vi "McP789A-Move-Server v0.80.vi"(5 "Initializing MCP":bool, 6 "Change Counter Position Manually":bool, 7 "error in":errorcluster, 8 "Unit":u8(ring)=1 items=["Point #", "nm", "eV", "meV", "cm-1"], 9 "New Position":dbl=600.0 min=0.0 max=100000.0 format="%.3f", 10 "Grating Density":enum16{"150", "300", "600", "1200", "1800"}(ring)=enum."1800") -> (0 "error out":errorcluster={"status"=TRUE, "code"=65, "source"="McP Timeout"}, 1 "Final Stepper Position":i32=-1000000, 2 "Final Wavelenth (nm)":dbl=222.0 format="%.2f", 3 "Final CounterReading":dbl=10000.0 min=0.0 max=26000.0 format="%.2f", 4 "Final Position":dbl=222.0 format="%.2f")   [LabVIEW 2020]
doc: "McPherson 789A-3 controller Vi to control McPherson 2075 spectrometer through serial port. If running directly, you need to initialize the serial port and the spectrometer. During this process, if the scan velocity returns to be 0, the program is suspended. You need to change the velocity manually to unblock."
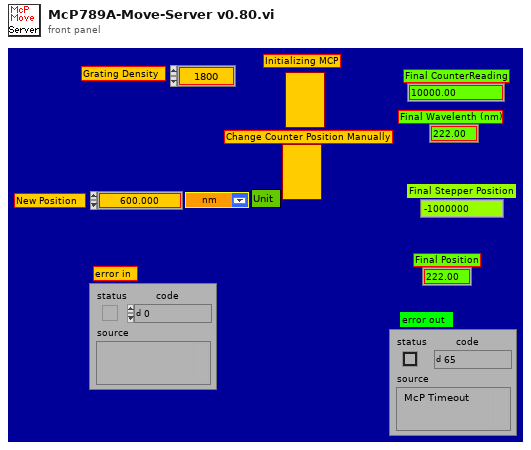
[diagram p1: front panel]
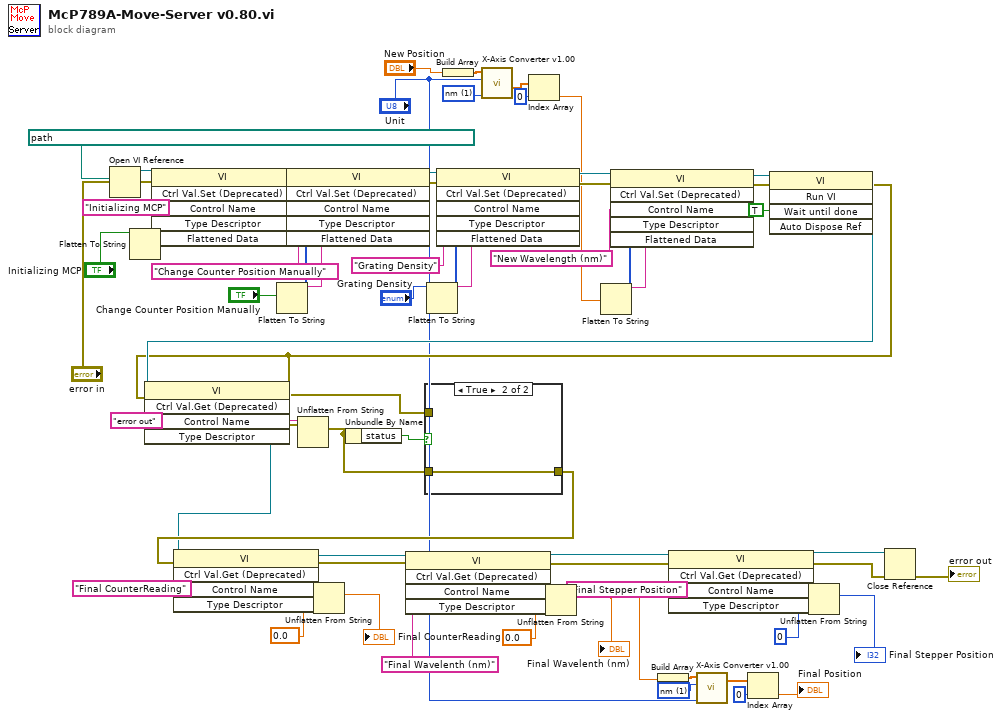
[diagram p0: block diagram]
diagram:
  w4 = 1 items=["Point #", "nm", "eV", "meV", "cm-1"] ("Old X-Axis Unit")
  w9 = 1 items=["Point #", "nm", "eV", "meV", "cm-1"] ("X-Axis Unit")
  n1 = Open VI Reference(vi path=path "/Optics2Mac/xwei Work/CCD Project/ƒ Subroutines/MCP/McP789A-Move-v0.80.vi") -> (vi reference=w66:refnum<vi>)  [unwired: 5 in, 1 out]
  n2 = Flatten To String(anything="Initializing MCP") -> (data string=w62:string, type string=w63:i16[])  [unwired: 3 in, 1 out]
  n3 = invoke class="VI" method="Ctrl Val.Set (Deprecated)"(reference=w66, error in="error in", "Control Name"="Initializing MCP", "Type Descriptor"=w63, "Flattened Data"=w62) -> (reference out=w60:refnum<vi>, error out=w59:errorcluster)  [unwired: 1 in, 4 out]
  n4 = Flatten To String(anything="Change Counter Position Manually") -> (data string=w56:string, type string=w57:i16[])  [unwired: 3 in, 1 out]
  n5 = invoke class="VI" method="Ctrl Val.Set (Deprecated)"(reference=w60, error in=w59, "Control Name"="Change Counter Position Manually", "Type Descriptor"=w57, "Flattened Data"=w56) -> (reference out=w52:refnum<vi>, error out=w51:errorcluster)  [unwired: 1 in, 4 out]
  n6 = Flatten To String(anything="Grating Density") -> (data string=w53:string, type string=w54:i16[])  [unwired: 3 in, 1 out]
  n7 = invoke class="VI" method="Ctrl Val.Set (Deprecated)"(reference=w52, error in=w51, "Control Name"="Grating Density", "Type Descriptor"=w54, "Flattened Data"=w53) -> (reference out=w45:refnum<vi>, error out=w44:errorcluster)  [unwired: 1 in, 4 out]
  n8 = Build Array("New Position") -> (w11:dbl[])
  n9 = call "X-Axis Converter v1.00.vi"("X-Axis Unit"=w9, "Old X-Axis Unit"="Unit", "X-Axis input"=w11) -> ("X-Axis Output"=w12:dbl[])  [unwired: 2 in, 3 out]
  n10 = Index Array(array=w12, index=0) -> (element=w8:dbl)
  n11 = Flatten To String(anything=w8) -> (data string=w48:string, type string=w49:i16[])  [unwired: 3 in, 1 out]
  n12 = invoke class="VI" method="Ctrl Val.Set (Deprecated)"(reference=w45, error in=w44, "Control Name"="New Wavelength (nm)", "Type Descriptor"=w49, "Flattened Data"=w48) -> (reference out=w43:refnum<vi>, error out=w42:errorcluster)  [unwired: 1 in, 4 out]
  n13 = invoke class="VI" method="Run VI"(reference=w43, error in=w42, "Wait until done"=TRUE) -> (reference out=w40:refnum<vi>, error out=w37:errorcluster)  [unwired: 2 in, 3 out]
  n14 = invoke class="VI" method="Ctrl Val.Get (Deprecated)"(reference=w40, error in=w37, "Control Name"="error out") -> (reference out=w14:refnum<vi>, error out=w34:errorcluster, "Get Control Value"=w38:string)  [unwired: 2 in, 2 out]
  n15 = Unflatten From String(type=w37, binary string=w38) -> (value=w35:errorcluster)  [unwired: 3 in, 2 out]
  n16 = Unbundle By Name(w35) -> ("status"=w36:bool)
  n17 = case shown="True" w36 {
    tunnel: [w68 w69] -> w33
    tunnel: w35 -> [_ w69]
    tunnel: w34 -> [w68 _]
    frame False {
    }
    frame True {
    }
  }
  n18 = invoke class="VI" method="Ctrl Val.Get (Deprecated)"(reference=w14, error in=w33, "Control Name"="Final CounterReading") -> (reference out=w22:refnum<vi>, error out=w21:errorcluster, "Get Control Value"=w31:string)  [unwired: 2 in, 2 out]
  n19 = Unflatten From String(type=0.0, binary string=w31) -> (value=→"Final CounterReading":dbl)  [unwired: 3 in, 2 out]
  n20 = invoke class="VI" method="Ctrl Val.Get (Deprecated)"(reference=w22, error in=w21, "Control Name"="Final Wavelenth (nm)") -> (reference out=w20:refnum<vi>, error out=w19:errorcluster, "Get Control Value"=w27:string)  [unwired: 2 in, 2 out]
  n21 = Unflatten From String(type=0.0, binary string=w27) -> (value=w3:dbl)  [unwired: 3 in, 2 out]
  "Final Wavelenth (nm)" <- w3
  n22 = Build Array(w3) -> (w5:dbl[])
  n23 = invoke class="VI" method="Ctrl Val.Get (Deprecated)"(reference=w20, error in=w19, "Control Name"="Final Stepper Position") -> (reference out=w17:refnum<vi>, error out=w16:errorcluster, "Get Control Value"=w24:string)  [unwired: 2 in, 2 out]
  n24 = call "X-Axis Converter v1.00.vi"("X-Axis Unit"="Unit", "Old X-Axis Unit"=w4, "X-Axis input"=w5) -> ("X-Axis Output"=w6:dbl[])  [unwired: 2 in, 3 out]
  n25 = Index Array(array=w6, index=0) -> (element=→"Final Position":dbl)
  n26 = Unflatten From String(type=0, binary string=w24) -> (value=→"Final Stepper Position":i32)  [unwired: 3 in, 2 out]
  n27 = Close Reference(reference=w17, error in (no error)=w16) -> (error out=→"error out":errorcluster)
